vi "Update Animation.vi"(11 "Asteroid in":refnum<class "Planet.lvclass">) -> (3 "Asteroid out":refnum<class "Planet.lvclass">)   [LabVIEW 2015]
uses:
  Planet.lvclass
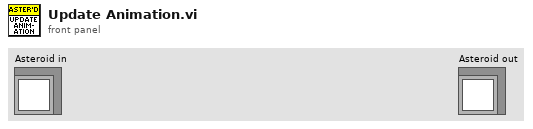
[diagram p1: front panel]
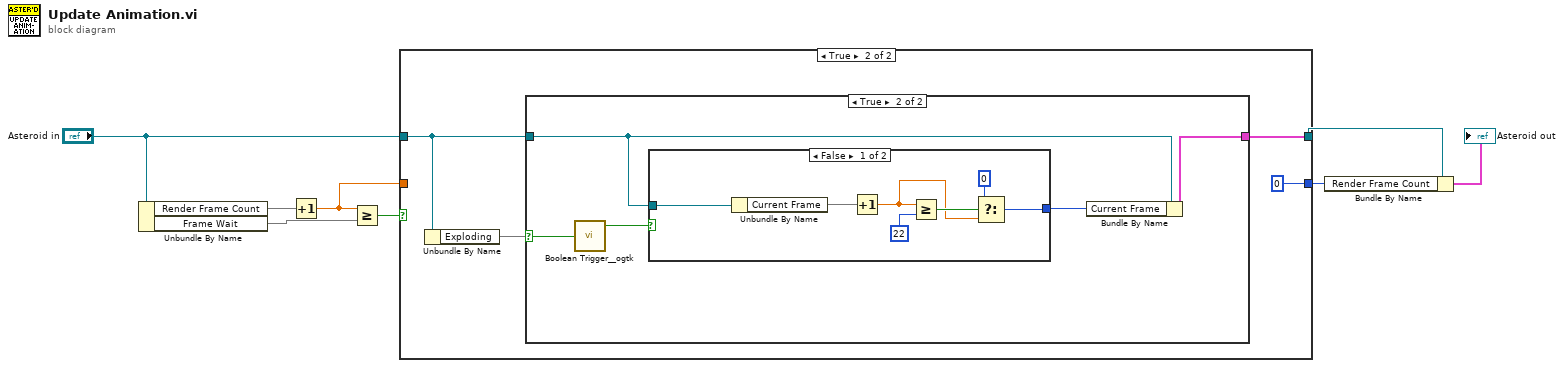
[diagram p0: block diagram]
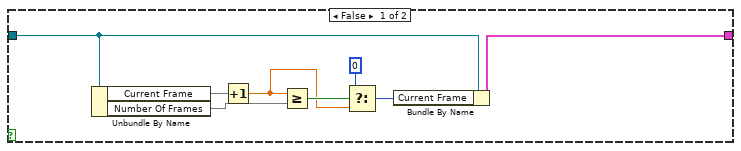
[diagram p3: hidden frame]
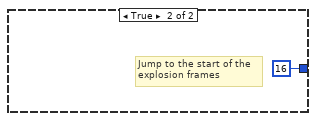
[diagram p4: hidden frame]
diagram:
  n1 = Unbundle By Name("Asteroid in") -> ("Render Frame Count"=w5, "Frame Wait"=w6)
  n2 = Increment(x=w5) -> (x+1=w8:dbl)
  n3 = Greater Or Equal?(x=w8, y=w6) -> (x >= y?=w7:bool)
  n4 = case shown="True" w7 {
    tunnel: [w10 w13] -> w1
    tunnel: "Asteroid in" -> [w10 w14]
    tunnel: w8 -> [w9 _]
    tunnel: [w9 0 ("Render Frame Count")] -> w3
    frame False {
    }
    frame True {
      n5 = Unbundle By Name(w14) -> ("Exploding"=w11)
      n6 = case shown="True" w11 {
        selector: w11 -> [_ w24]
        tunnel: [w22 w26] -> w13
        tunnel: w14 -> [w15 w25]
        frame False {
          n7 = Unbundle By Name(w15) -> ("Current Frame"=w21, "Number Of Frames"=w19)
          n8 = Increment(x=w21) -> (x+1=w16:dbl)
          n9 = Greater Or Equal?(x=w16, y=w19) -> (x >= y?=w18:bool)
          n10 = Select(t=0, s=w18, f=w16) -> (s? t:f=w20:i32)
          n11 = Bundle By Name(cluster=w15, "Current Frame"=w20) -> (w22:cluster{})
        }
        frame True {
          n12 = call <userlib>:"Boolean Trigger__ogtk.vi"("Boolean Input"=w24) -> ("Rising Edge"=w23:bool)  [unwired: 1 in, 1 out]
          n13 = case shown="False" w23 {
            tunnel: [w33 16 ("t")] -> w27
            tunnel: w25 -> [w28 _]
            frame False {
              n14 = Unbundle By Name(w28) -> ("Current Frame"=w34)
              n15 = Increment(x=w34) -> (x+1=w30:dbl)
              n16 = Greater Or Equal?(x=w30, y=22) -> (x >= y?=w32:bool)
              n17 = Select(t=0, s=w32, f=w30) -> (s? t:f=w33:i32)
            }
            frame True {
              # "Jump to the start of the explosion frames"
            }
          }
          n18 = Bundle By Name(cluster=w25, "Current Frame"=w27) -> (w26:cluster{})
        }
      }
    }
  }
  n19 = Bundle By Name(cluster=w1, "Render Frame Count"=w3) -> (→"Asteroid out":cluster{})
